vi "Timer FGV for Delay.vi"(10 "Reset":bool, 11 "Time Target (ticks)":u32) -> (2 "Time Reached?":bool, 3 "Time elapsed (ticks)":u32)   [LabVIEW 2014]
doc: "Set a time target (ticks) and it will tell you if the time has been reached.\nThis VI auto resets the time target.\nCompatible with SCTL."
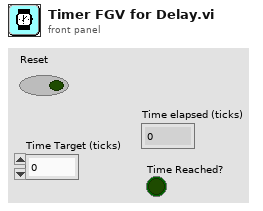
[diagram p1: front panel]
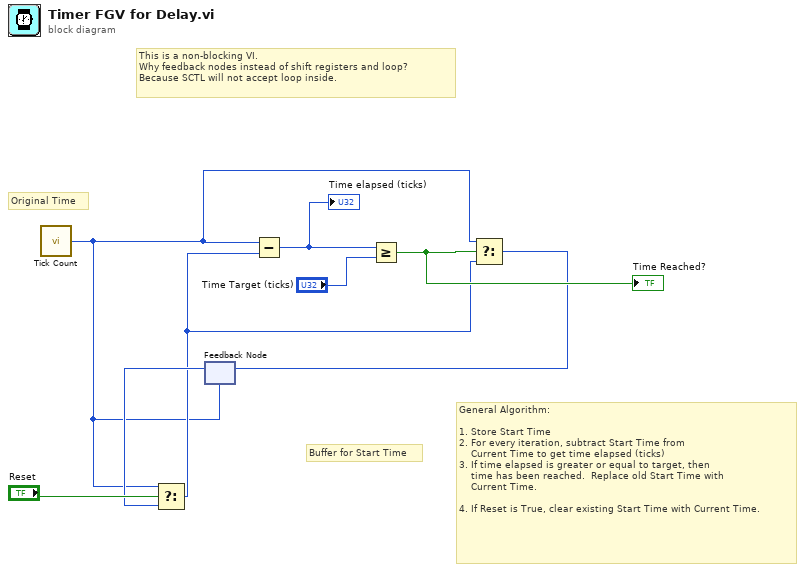
[diagram p0: block diagram]
diagram:
  # "Buffer for Start Time"
  # "This is a non-blocking VI.\nWhy feedback nodes instead of shift registers and loop?\nBecause SCTL will not accept loop inside."
  # "Original Time"
  # "General Algorithm:\n\n1. Store Start Time\n2. For every iteration, subtract Start Time from \n    Current Time to get time elapsed (ticks)\n3. If time elapsed is greater or equal to target, then\n    time has been reached.  Replace old Start Time with\n    Current Time.\n\n4. If Reset is True, clear existing Start Time with Current Time."
  n1 = call "Tick Count"() -> ("Tick Count(Ticks)"=w1:u32)
  n2 = feedback #1(w1) -> (w3:u32)
  n3 = Select(t=w1, s="Reset", f=w3) -> (s? t:f=w2:u32)
  n4 = Subtract(x=w1, y=w2) -> (x-y=w7:u32)
  "Time elapsed (ticks)" <- w7
  n5 = Greater Or Equal?(x=w7, y="Time Target (ticks)") -> (x >= y?=w8:bool)
  "Time Reached?" <- w8
  n6 = Select(t=w1, s=w8, f=w2) -> (s? t:f=w5:u32)
  n7 = feedback-in #1(w5) -> ()
